vi "Read Text.vi"(6 "error in":errorcluster, 8 "timeout ms (5000)":i32=5000, 9 "RawSocket Handler in":refnum<class "RawSocket TCP Handler.lvclass">) -> (0 "error out":errorcluster, 1 "String":string, 3 "RawSocket Handler out":refnum<class "RawSocket TCP Handler.lvclass">)   [LabVIEW 2020, in "wamplv.lvlib" / "RawSocket TCP Handler.lvclass"]
uses:
  RawSocket TCP Handler.lvclass
  RawSocket TCP Handler.lvclass/RawSocket TCP Handler.ctl
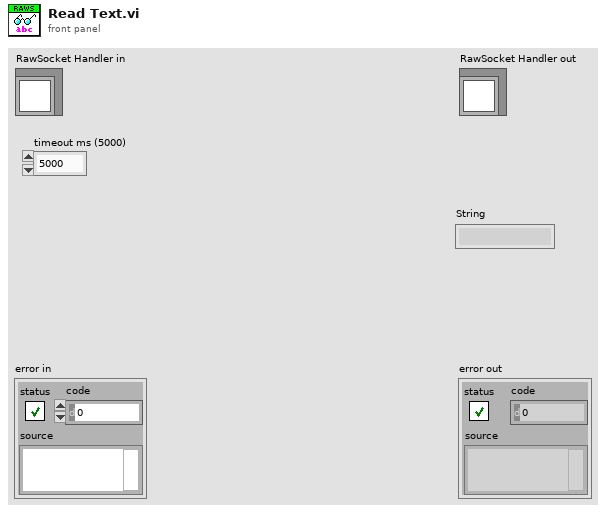
[diagram p1: front panel]
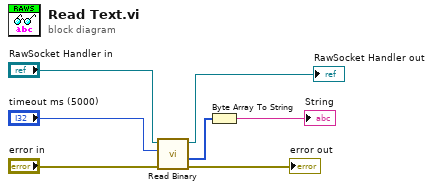
[diagram p0: block diagram]
diagram:
  n1 = call-dynamic "Read Binary.vi"("error in (no error)"="error in", "timeout ms (5000)"="timeout ms (5000)", "RawSocket TCP Handler in"="RawSocket Handler in") -> ("error out"=→"error out":errorcluster, "Bytes"=w2:u8[], "RawSocket TCP Handler out"=→"RawSocket Handler out":refnum<class "RawSocket TCP Handler.lvclass">)  [unwired: 4 in]
  n2 = Byte Array To String(unsigned byte array=w2) -> (string=→"String":string)
